vi "Acroname_All_Ports_Disable.vi"(8 "error in (no error)":errorcluster) -> (0 "error out":errorcluster, 2 "Ports Failed":i32[](array[numeric]))   [LabVIEW 2025]
uses:
  02def416-1e0c-4ca4-a1f8-c324895dea06.vi
  BrainStem2_LabVIEW_Library.lvlib
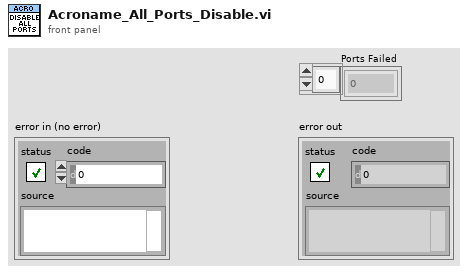
[diagram p1: front panel]
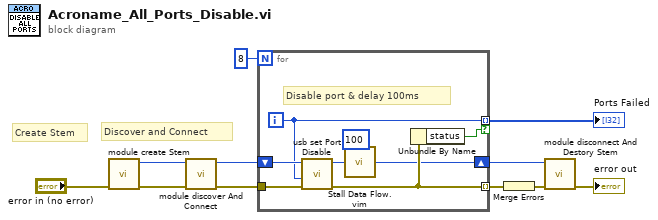
[diagram p0: block diagram]
diagram:
  # "Discover and Connect"
  # "Create Stem"
  n1 = call "module create Stem.vi"("error in (no error)"="error in (no error)") -> ("error out"=w7:errorcluster, "id out"=w8:u32)  [unwired: 8 in, 1 out]
  n2 = call "module discover And Connect.vi"("error in (no error)"=w7, "id"=w8) -> ("error out"=w5:errorcluster, "id out"=w4:u32)  [unwired: 7 in, 1 out]
  n3 = for {
    N: 8 -> [_]
    tunnel: [w12] -> w10 mode=indexing if=w19
    tunnel: [w14] -> w9 mode=indexing
    tunnel: w5 -> [w16]
    shift-right: [w13] -> w1
    shift-left: w4 -> [w15]
    i -> [w12]
    # "Disable port & delay 100ms"
    n4 = call "usb set Port Disable.vi"("error in (no error)"=w16, "channel"=w12, "id"=w15) -> ("error out"=w14:errorcluster, "id out"=w18:u32)  [unwired: 6 in, 1 out]
    n5 = call "Stall Data Flow.vim"("value in"=w18, "milliseconds to wait"=100) -> ("value out"=w13:u32)  [unwired: 1 out]
    n6 = Unbundle By Name(w14) -> ("status"=w19:bool)
  }
  "Ports Failed" <- w10
  n7 = Merge Errors(w9) -> (w3:errorcluster)
  n8 = call "module disconnect And Destory Stem.vi"("error in (no error)"=w3, "id"=w1) -> ("error out"=→"error out":errorcluster)  [unwired: 7 in, 2 out]
